vi "SubStage_OpenExcelandMakeVisible.vi"(2 "error in (no error)":errorcluster, 3 "Visible Boolean":bool=TRUE) -> (0 "error out":errorcluster, 1 "Excel._Application":refnum<k7>)   [LabVIEW 2015]
doc: "This VI opens Excel by creating an Automation Refnum for the Excel.Application object. Next it sets the \"Visible\" property to True/False depending on the Visible input."
panel:
  in  "Excel._Application":refnum<k7>
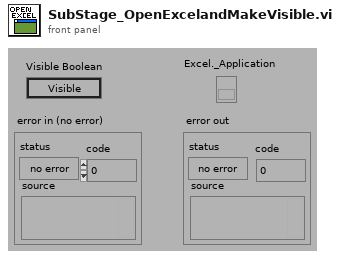
[diagram p1: front panel]
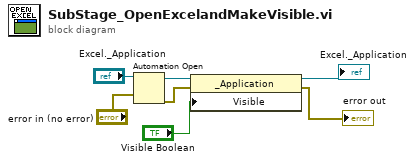
[diagram p0: block diagram]
diagram:
  n1 = Automation Open(error in (no error)="error in (no error)", Automation Refnum="Excel._Application") -> (Automation Refnum=w4:refnum<k7>, error out=w3:errorcluster)  [unwired: 2 in]
  n2 = property class="_Application"(reference=w4, error in=w3, "Visible"="Visible Boolean") -> (reference out=→"Excel._Application":refnum<k7>, error out=→"error out":errorcluster)
